vi "Get Names of All Running VIs.vi"(2 "error in (no error)":errorcluster) -> (0 "error out":errorcluster, 1 "Item Names":string[](array[string]))   [LabVIEW 2009]
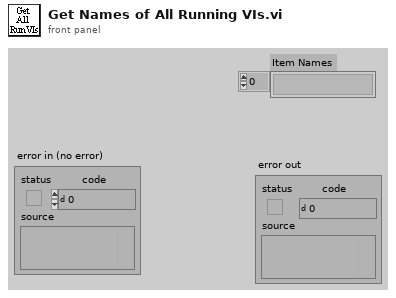
[diagram p1: front panel]
types:
  T1 = enum32{"Bad", "Idle", "Run top level", "Running"}
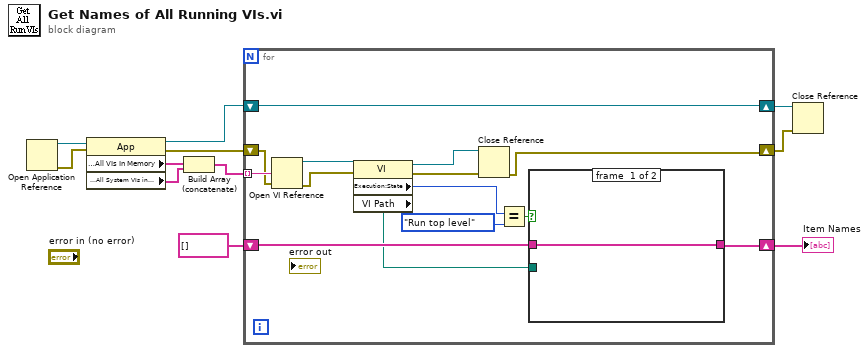
[diagram p0: block diagram]
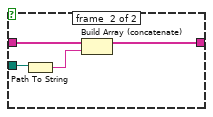
[diagram p2: hidden frame]
diagram:
  n1 = Open Application Reference() -> (0:w2:errorcluster, 3:w1:refnum<vi>)  [unwired: 4 in]
  n2 = property class="App"(reference=w1, error in=w2) -> (reference out=w6:refnum<vi>, error out=w10:errorcluster, "Application:All VIs In Memory"=w7:string[], "Application:All System VIs in Memory"=w8:string[])
  n3 = Build Array (concatenate)(w7, w8) -> (w9:string[])
  n4 = for {
    tunnel: w9 -> [w18] mode=indexing
    shift-right: [w19] -> w4
    shift-left: string[] [] ("App.AllVIs") -> [w20]
    shift-right: [w15] -> w5
    shift-left: w6 -> [w15]
    shift-right: [w13] -> w11
    shift-left: w10 -> [w14]
    n5 = Open VI Reference(vi path=w18, error in (no error)=w14) -> (vi reference=w25:refnum<vi>, error out=w24:errorcluster)  [unwired: 4 in]
    n6 = property class="VI"(reference=w25, error in=w24) -> (reference out=w17:refnum<vi>, error out=w16:errorcluster, "Execution:State"=w23:T1, "VI Path"=w12:path)
    n7 = Close Reference(reference=w17, error in (no error)=w16) -> (error out=w13:errorcluster)
    n8 = Equal?(x=w23, y=T1."Run top level" ("Exec.State")) -> (x = y?=w21:bool)
    n9 = case shown="True" w21 {
      tunnel: [w26 w29] -> w19
      tunnel: w20 -> [w26 w30]
      tunnel: w12 -> [_ w28]
      frame #0 {
      }
      frame #1 {
        n10 = Path To String(path=w28) -> (string=w27:string)
        n11 = Build Array (concatenate)(w30, w27) -> (w29:string[])
      }
    }
  }
  "Item Names" <- w4
  n12 = Close Reference(reference=w5, error in (no error)=w11) -> ()  [unwired: 1 out]
